vi "Get Author Name.vi"(8 "error in (no error)":errorcluster, 11 "MyMouse in":refnum<class "MyMouse.lvclass">) -> (0 "error out":errorcluster, 2 "Author":string, 3 "MyMouse out":refnum<class "MyMouse.lvclass">)   [LabVIEW 2020, in "Mouse.lvlib" / "MyMouse.lvclass"]
uses:
  MyMouse.lvclass
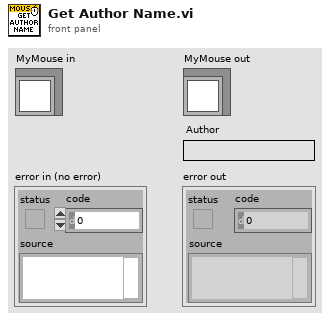
[diagram p1: front panel]
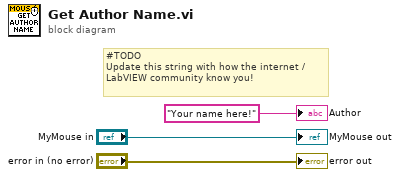
[diagram p0: block diagram]
diagram:
  # "#TODO\nUpdate this string with how the internet / LabVIEW community know you!"
  "error out" <- "error in (no error)"
  "MyMouse out" <- "MyMouse in"
  "Author" <- "Your name here!" ("Author")
